vi "Display New Line.vi"(8 "error in (no error)":errorcluster, 11 "Logger Normal in":refnum<class "Logger Normal.lvclass">) -> (0 "error out":errorcluster, 3 "Logger Normal out":refnum<class "Logger Normal.lvclass">)   [LabVIEW 2020, in "Logger Normal.lvlib" / "Logger Normal.lvclass"]
uses:
  Logger Normal.lvclass
  <vilib>/Utility/miscctls.llb/LVRowAndColumnUnsignedTypeDef.ctl
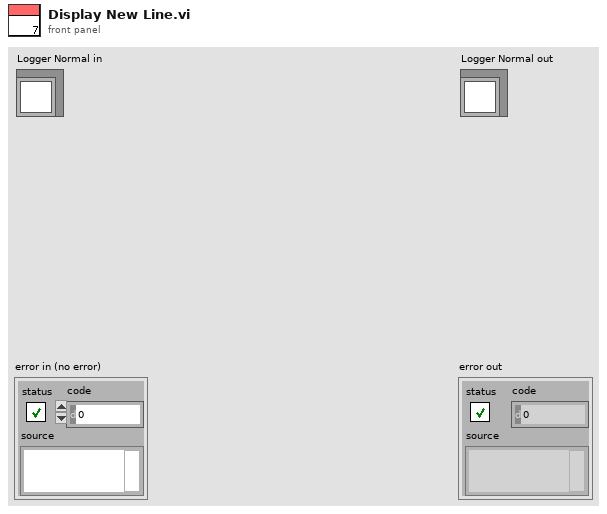
[diagram p1: front panel]
types:
  T1 = typedef "LVRowAndColumnUnsignedTypeDef.ctl" = cluster{"Row":u32, "Column":u32}
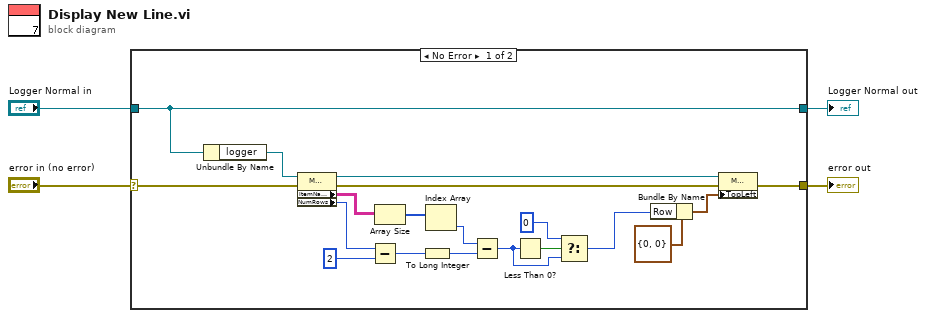
[diagram p0: block diagram]
diagram:
  n1 = case shown="No Error" "error in (no error)" {
    selector: "error in (no error)" -> [w19 w25]
    tunnel: [w22 w25] -> w3
    tunnel: [w23 w24] -> w1
    tunnel: "Logger Normal in" -> [w23 w24]
    frame No Error {
      n2 = Unbundle By Name(w23) -> ("logger"=w18:refnum<vi>)
      n3 = property class="MCListbox (strict)"(reference=w18, error in=w19) -> (reference out=w6:refnum<vi>, error out=w11:errorcluster, "ItemNames"=w17:string[][], "NumRows"=w15:u32)
      n4 = Subtract(x=w15, y=u32 2) -> (x-y=w13:u32)
      n5 = Array Size(array=w17) -> (size(s)=w16:i32[])
      n6 = To Long Integer(number=w13) -> (32bit integer=w5:i32)
      n7 = Index Array(array=w16) -> (element=w12:i32)  [unwired: 1 in]
      n8 = Subtract(x=w12, y=w5) -> (x-y=w8:i32)
      n9 = Less Than 0?(x=w8) -> (x < 0?=w10:bool)
      n10 = Select(t=0, s=w10, f=w8) -> (s? t:f=w7:i32)
      n11 = Bundle By Name(cluster=T1 {"Row"=0, "Column"=0} ("Top Left Visible Cell"), "Row"=w7) -> (w20:T1)
      n12 = property class="MCListbox (strict)"(reference=w6, error in=w11, "TopLeft"=w20) -> (error out=w22:errorcluster)  [unwired: 1 out]
    }
    frame Error {
    }
  }
  "error out" <- w3
  "Logger Normal out" <- w1
